vi "BioFeedback11(SingleBarBiofeedback).vi"(0 "UI Data Right":path=path "C:/Users/Tinggroup/Desktop/VRMuscleActivationVisualizer/VRBiofeedback_v2/assets/RightEMGData.txt", 7 "Frames Per Second":dbl=30.0, 9 "Start Trial":bool, 11 "End Trial":bool, 12 "Data Directory":path, 13 "File Name":string, 14 "Extension":string="_EMG.txt") -> ()   [LabVIEW 2016]
uses:
  <vilib>/Utility/error.llb/DialogType.ctl
  <vilib>/Analysis/5stat.llb/RMS (DBL).vi
  <vilib>/Waveform/WDTOps.llb/WDT Append Waveforms DBL.vi
  <vilib>/Utility/file.llb/Write Delimited Spreadsheet (string).vi
  <vilib>/Waveform/WDTFileIO.llb/Export Waveforms To Spreadsheet File (1D).vi
  <vilib>/Analysis/NI_AALPro.lvlib
panel:
  out "Trial Data Column Headers":string[](array[string])
  in  "TrialDataRowHeaders":string[](array[string])
  out "GetMaxStartTime":timestamp
  in  "SecondsToAcquireMax":dbl=10.0
  in  "NumberOfMaximumsInAverage":dbl=3.0
  in  "CurrentMaxIndex":dbl
  out "SignalsAvgMaxArray":dbl[](array[numeric])
  out "SignalMaxArray":dbl[][](array[numeric])
  in  "%StdDevIndex":dbl=5.0
  in  "Mean%Index":dbl=4.0
  in  "StdDevIndex":dbl=3.0
  in  "MeanIndex":dbl=2.0
  in  "MaxIndex":dbl=1.0
  in  "MinIndex":dbl
  out "Stability Data":dbl[][](array[numeric])
  out "2d target":cluster{dbl[], dbl[]}[](graph)
  out "trialFilteredData":waveform(dbl)[](array[waveform])
  out "filteredWaveforms":waveform(dbl)[](array[waveform])
  in  "UI Ampl Error Path":path=path "C:/Users/Tinggroup/Desktop/VRMuscleActivationVisualizer/VRBiofeedback_v2/assets/BiofeedbackAmplitudeError.txt"
  in  "UI L/R Error Path":path=path "C:/Users/Tinggroup/Desktop/VRMuscleActivationVisualizer/VRBiofeedback_v2/assets/BiofeedbackLRError.txt"
  out "LeftPercentActivation":dbl
  out "RightPercentActivation":dbl
  out "LeftMovingAvg":dbl
  out "RightMovingAvg":dbl
  in  "AutoAnalyzeStablity":bool
  out "PointCluster":cluster{dbl[], dbl[]}
  out "combined y value":dbl
  out "Acquiring Max":bool
  in  "resetMax":bool
  in  "startGetMax":bool
  in  "Right Max":dbl
  in  "Left Max":dbl
  in  "Amplitude Error":dbl
  in  "L/R error":dbl
  in  "RightSignalB":dbl=6.0
  in  "RightSignalA":dbl=5.0
  in  "LefftSignalB":dbl=2.0
  in  "LeftSignalA":dbl=1.0
  out "Aggregate 8":waveform(dbl)[](array[waveform])
  in  "UI Data Left":path=path "C:/Users/Tinggroup/Desktop/VRMuscleActivationVisualizer/VRBiofeedback_v2/assets/LeftEMGData.txt"
  in  "EMG Input Device\nProduct Type":string="USB-6009"
  out "DispLeftMovingAvg":dbl(slide) caption="Left" max=1.0 scale=0.0..100.0
  out "DispRightMovingAvg":dbl(slide) caption="Right" max=0.01 scale=0.0..100.0
  out "RMS Right":dbl(graph)
  out "RMS Left":dbl(graph)
  out "RMS 8":dbl(graph)
  out "RMS 7":dbl(graph)
  out "RMS 6":dbl(graph)
  out "RMS 5":dbl(graph)
  out "RMS 4":dbl(graph)
  out "RMS 3":dbl(graph)
  out "RMS 2":dbl(graph)
  out "RMS 1":dbl(graph)
  out "Aggregate7":waveform(dbl)[](array[waveform])
  out "Aggregate6":waveform(dbl)[](array[waveform])
  out "Aggregate5":waveform(dbl)[](array[waveform])
  out "Aggregate4":waveform(dbl)[](array[waveform])
  out "Aggregate3":waveform(dbl)[](array[waveform])
  out "Aggregate2":waveform(dbl)[](array[waveform])
  out "Aggregate1":waveform(dbl)[](array[waveform])
  out "Wfm8":waveform(dbl)(graph)
  out "Wfm7":waveform(dbl)(graph)
  out "Wfm6":waveform(dbl)(graph)
  out "Wfm5":waveform(dbl)(graph)
  out "Wfm4":waveform(dbl)(graph)
  out "Wfm3":waveform(dbl)(graph)
  out "Wfm2":waveform(dbl)(graph)
  out "Wfm1":waveform(dbl)(graph)
  out "Trial Raw Waveforms":waveform(dbl)[](graph)
  in  "UI Percent Path":path=path "C:/Users/Tinggroup/Desktop/VRMuscleActivationVisualizer/VRBiofeedback_v2/assets/BiofeedbackTargetPercentage.txt"
  in  "Target Percentage":dbl=10.0
  out "Trial In Progress":bool
  in  "Lower Cut-Off":dbl=20.0
  in  "Upper Cut-Off":dbl=300.0
  out "raw data":dynamicdata(graph)
  out "Bufffer Index":dbl
  out "Frames in Buffer":dbl
  out "Samples per frame":dbl
  out "Reset Data Acquisition\nAnd UI Updating":bool=TRUE
  in  "Moving Average Length (s)":dbl=0.5
  in  "Sample rate (Hz)":dbl=2000.0
  in  "End Program":bool
  # "Saving Trial Data"
  # "Set Target and Box Size"
  # "Set Scale"
  # "These scale the thermometers and are used in mean calculation"
  # "Analyze Stability of Displayed Data"
  # "Auto Analyze Stability begins calculating stability\nAs soon as dot enters the target zone and stops \nonce the dot leaves the target zone (Not Yet Implemented)"
  # "Channels used in Display"
  # "Filter and Process Parameters"
  # "Changes are made instantly and cause moving average to reset to zero"
  # "for testing smaller sample\nsizes in getting max/min\nand stability data"
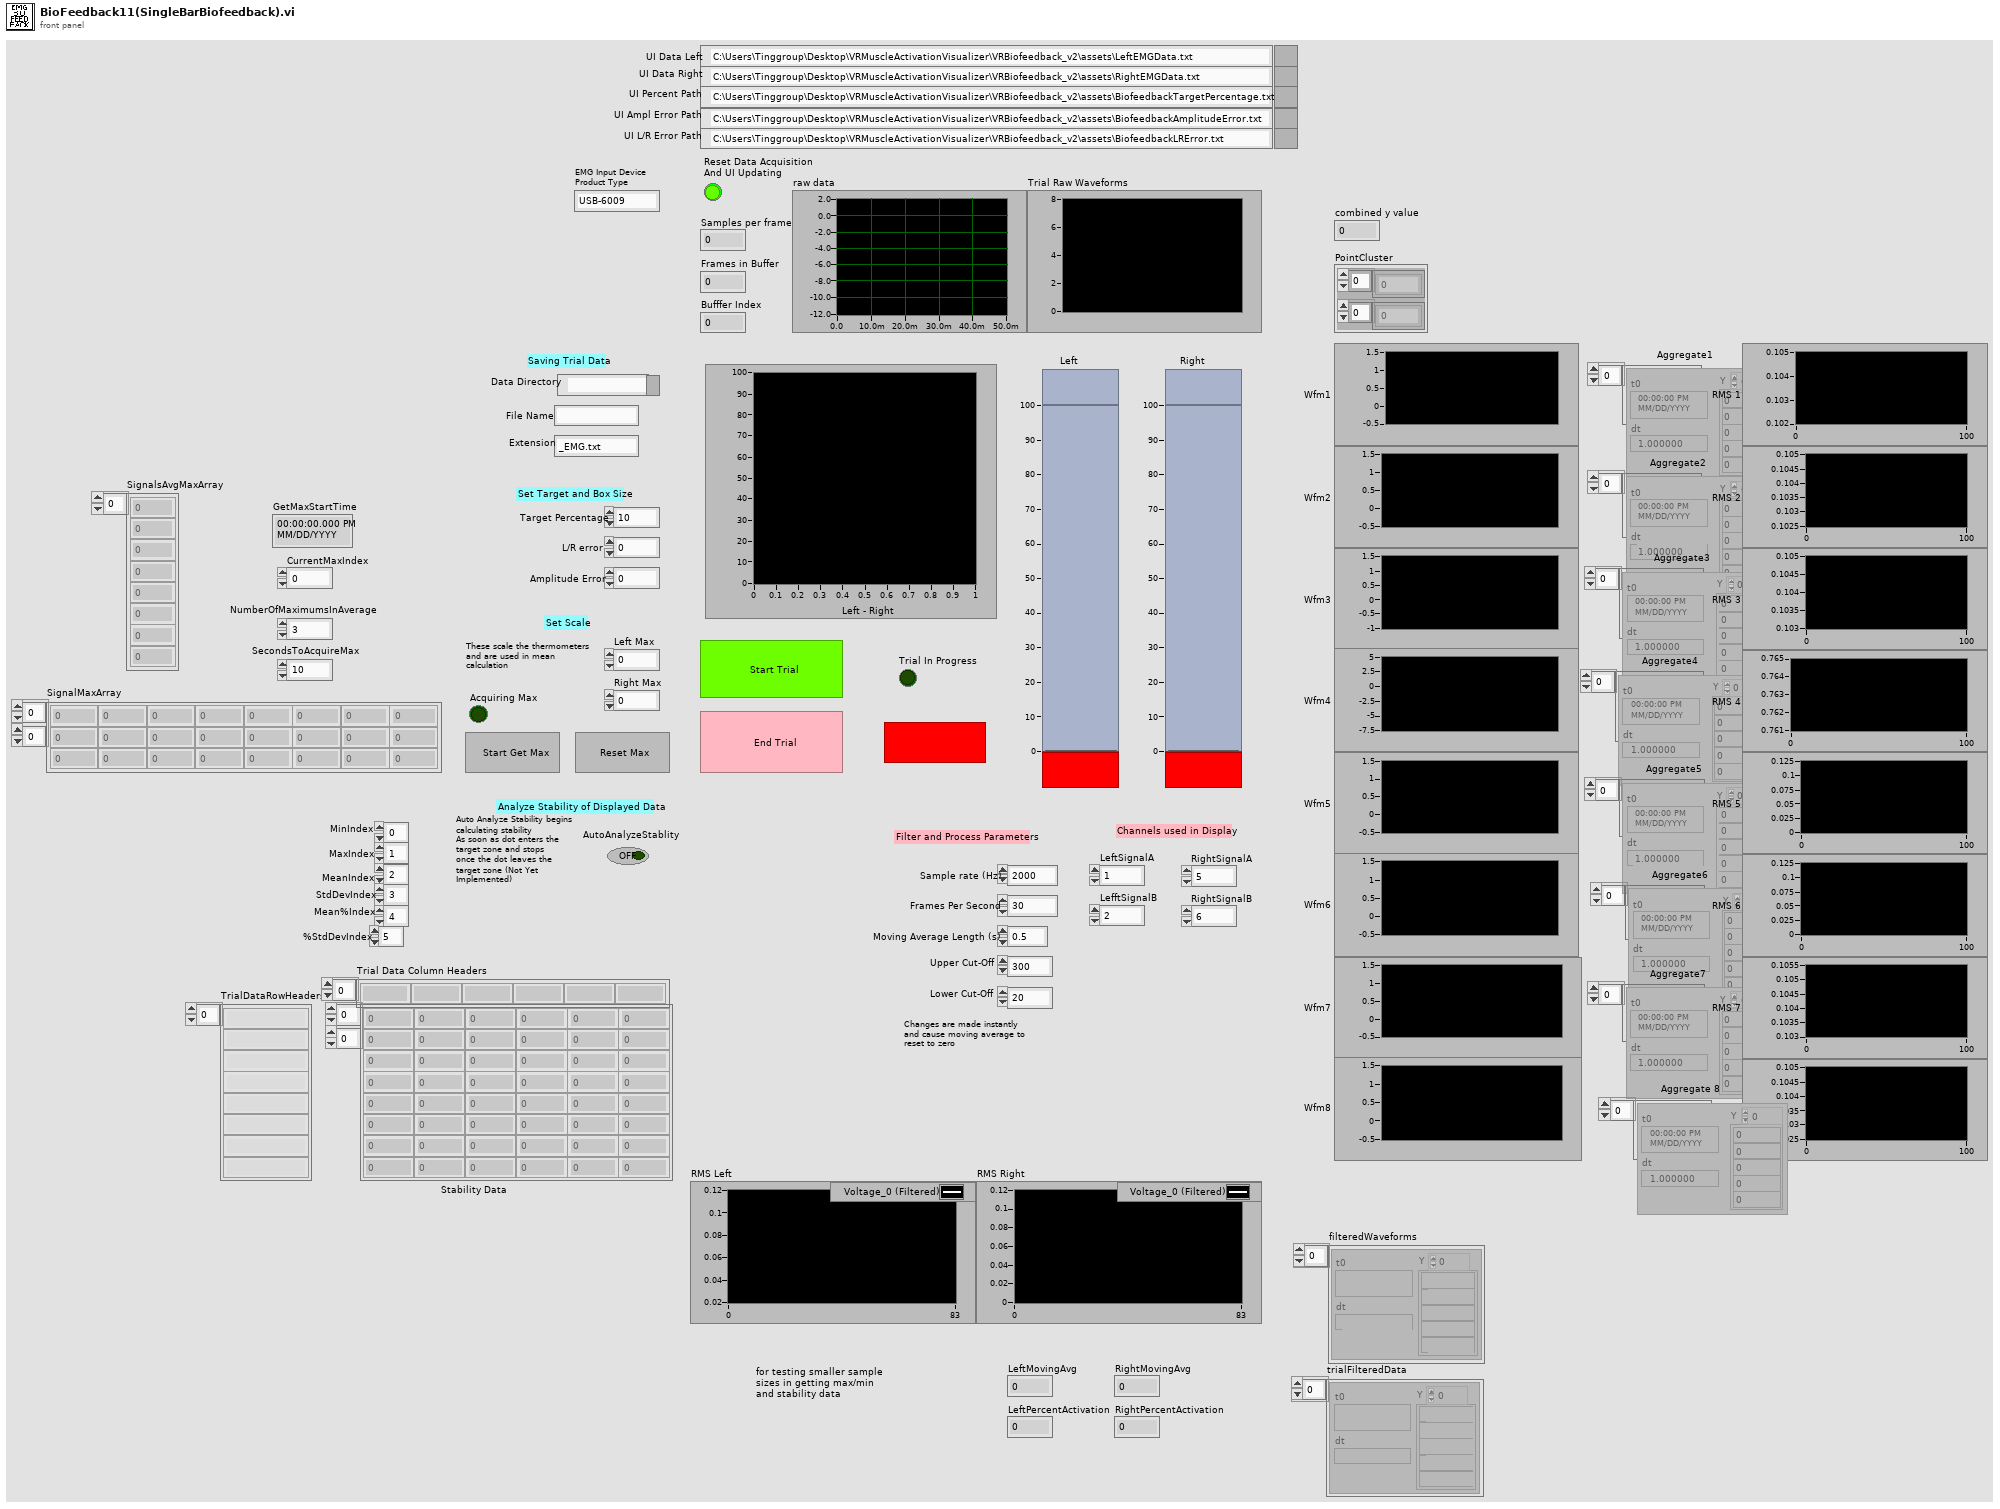
[diagram p1: front panel]
types:
  T1 = typedef "DialogType.ctl" = u16
  T2 = typedef "WaveformArrayControl.ctl" = waveform(dbl)[]
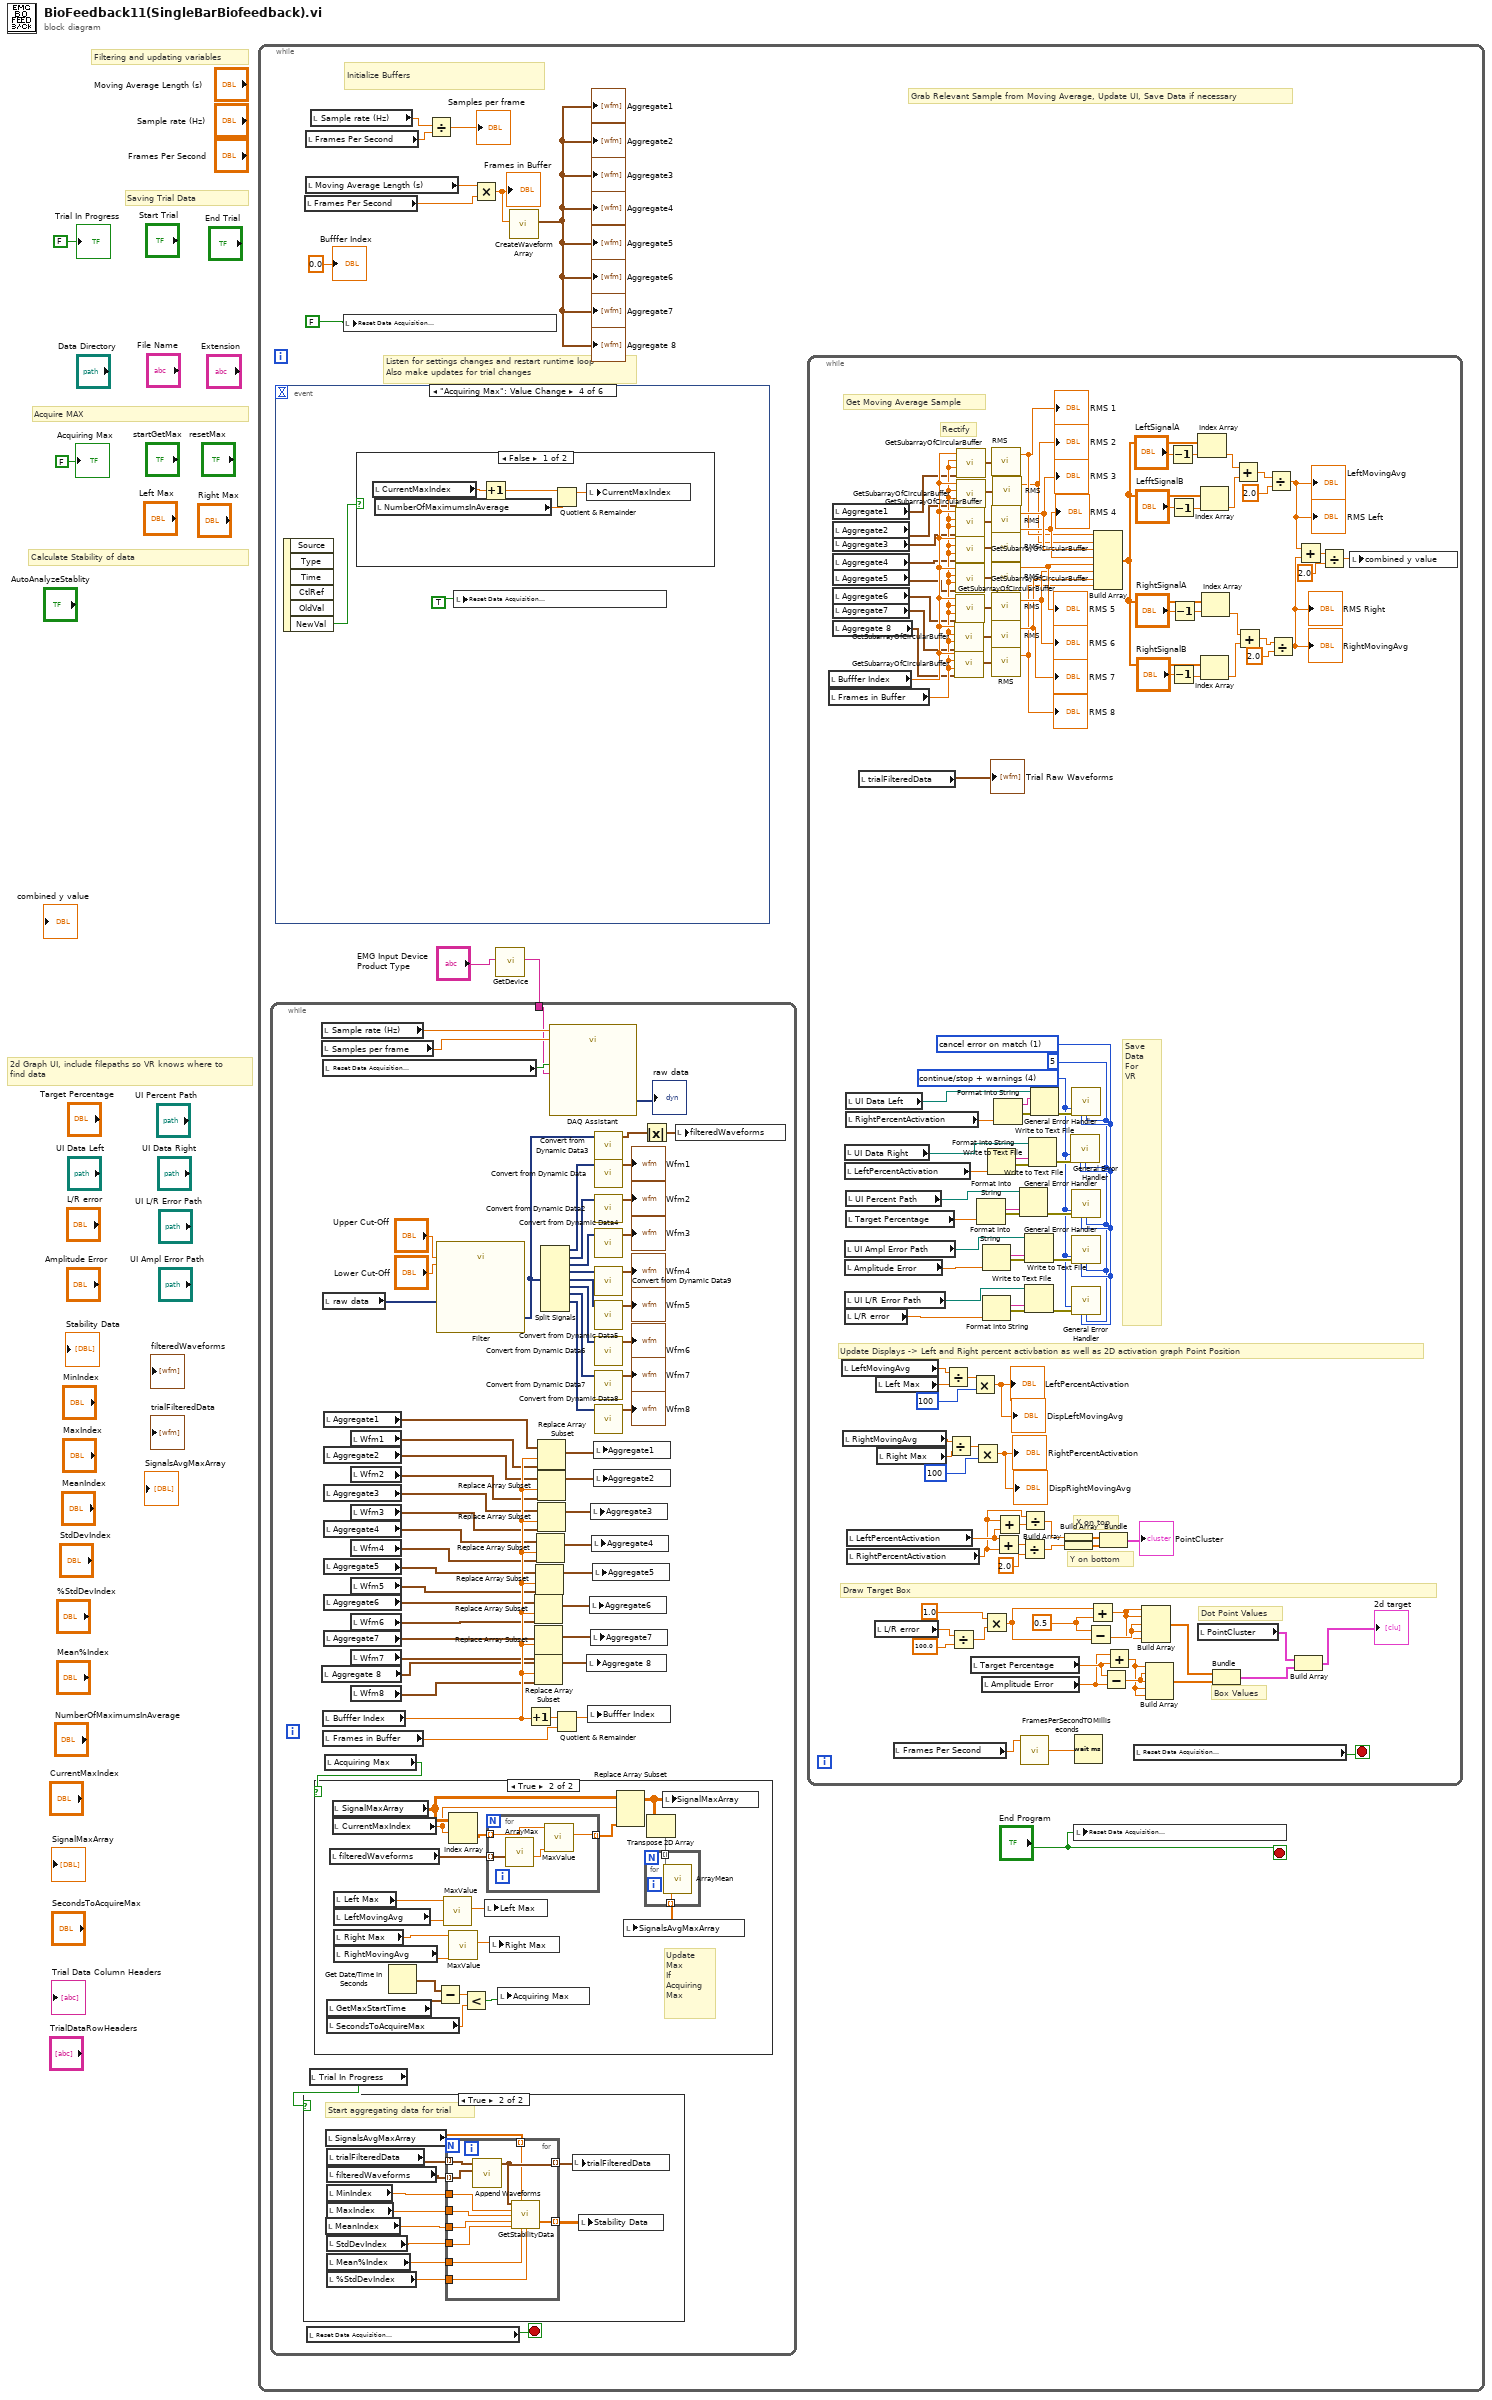
[diagram p0: block diagram]
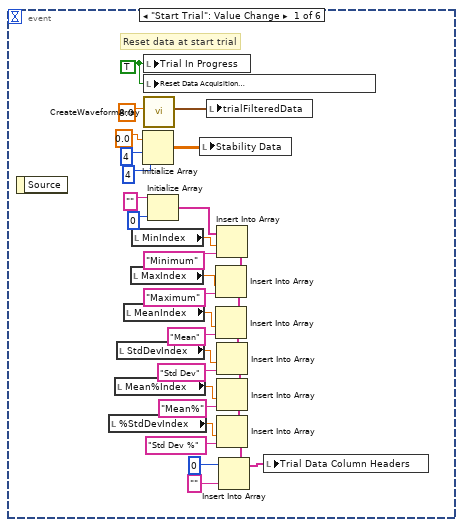
[diagram p2: hidden frame]
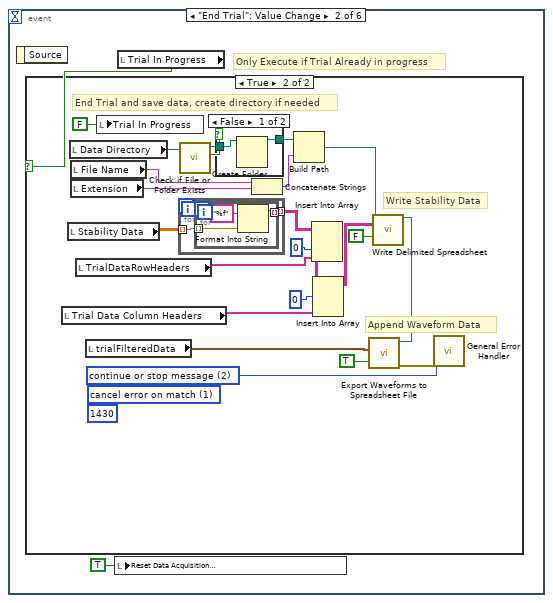
[diagram p3: hidden frame]
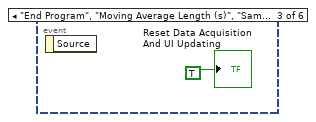
[diagram p6: hidden frame]
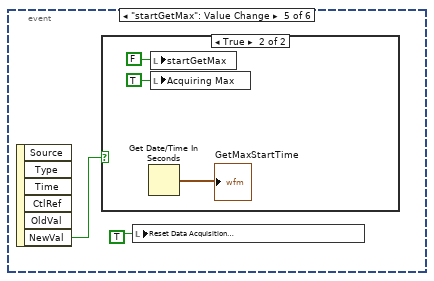
[diagram p8: hidden frame]
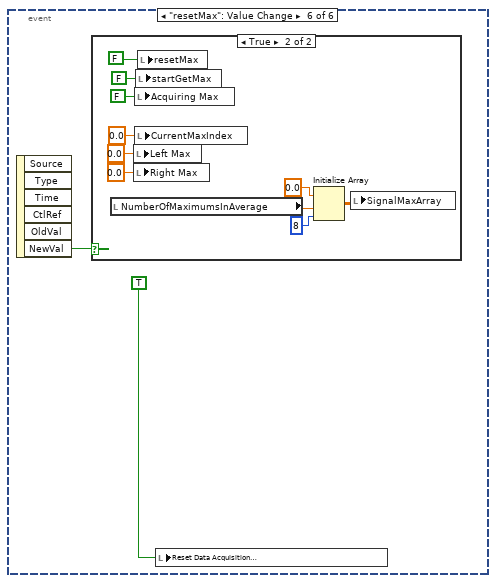
[diagram p10: hidden frame]
diagram:
  # "Calculate Stability of data"
  # "Acquire MAX"
  # "Filtering and updating variables"
  # "Saving Trial Data"
  # "2d Graph UI, include filepaths so VR knows where to find data"
  n1 = while {
    stop <- "End Program" stop-if-true
    # "Grab Relevant Sample from Moving Average, Update UI, Save Data if necessary"
    # "Initialize Buffers"
    # "Listen for settings changes and restart runtime loop\nAlso make updates for trial changes"
    n2 = event shown="[3] \"Acquiring Max\": Value Change" {
      selector: _ -> [_ _ _ _ _ _]
      dyn-events: _ -> [_ _ _ _ _ _]
      timeout: _ -> [_ _ _ _ _ _]
      event "Start Trial": Value Change {
        w45 = TRUE ("Trial In Progress")
        # "Reset data at start trial"
        n3 = event-data() -> ()  [unwired: 1 in, 1 out]
        n4 = local read "%StdDevIndex"() -> (w21:dbl)
        n5 = local read "Mean%Index"() -> (w22:dbl)
        n6 = local read "StdDevIndex"() -> (w26:dbl)
        n7 = local read "MeanIndex"() -> (w30:dbl)
        n8 = local read "MaxIndex"() -> (w33:dbl)
        n9 = local read "MinIndex"() -> (w35:dbl)
        n10 = Initialize Array(0.0 ("element"), 4 ("dimension size"), 4 ("dimension size")) -> (w39:dbl[][])
        n11 = local write "Trial In Progress"(w45) -> ()
        n12 = local write "Reset Data Acquisition\nAnd UI Updating"(w45) -> ()
        n13 = call "CreateWaveformArray.vi"("bufferSize"=8.0) -> ("initialized array"=w44:waveform(dbl)[])  [unwired: 5 in, 1 out]
        n14 = Initialize Array("", 0 ("dimension size")) -> (w34:string[])
        n15 = local write "Stability Data"(w39) -> ()
        n16 = local write "trialFilteredData"(w44) -> ()
        n17 = Insert Into Array(array=w34, index=w35, new element="Minimum" ("new element/subarray")) -> (w31:string[])
        n18 = Insert Into Array(array=w31, index=w33, new element="Maximum" ("new element/subarray")) -> (w28:string[])
        n19 = Insert Into Array(array=w28, index=w30, new element="Mean" ("new element/subarray")) -> (w25:string[])
        n20 = Insert Into Array(array=w25, index=w26, new element="Std Dev" ("new element/subarray")) -> (w23:string[])
        n21 = Insert Into Array(array=w23, index=w22, new element="Mean%" ("new element/subarray")) -> (w19:string[])
        n22 = Insert Into Array(array=w19, index=w21, new element="Std Dev %" ("new element/subarray")) -> (w16:string[])
        n23 = Insert Into Array(array=w16, index=0, new element="" ("new element/subarray")) -> (w17:string[])
        n24 = local write "Trial Data Column Headers"(w17) -> ()
      }
      event "End Trial": Value Change {
        # "Only Execute if Trial Already in progress"
        n25 = event-data() -> ()  [unwired: 1 in, 1 out]
        n26 = local write "Reset Data Acquisition\nAnd UI Updating"(TRUE ("Reset Data Acquisition\nAnd UI Updating")) -> ()
        n27 = local read "Trial In Progress"() -> (w47:bool)
        n28 = case shown="True" w47 {
          frame False {
          }
          frame True {
            w66 = T1 2 items=["no dialog", "OK message", "continue or stop message", "OK message + warnings", "continue/stop + warnings"] ("type of dialog (OK msg:1)")
            (unwired) 1 items=["no exception", "cancel error on match", "set error on match"] ("[exception action] (none:0)")
            (unwired) 1430 ("[exception code]")
            # "Append Waveform Data"
            # "Write Stability Data"
            # "End Trial and save data, create directory if needed"
            n29 = local read "Trial Data Column Headers"() -> (w54:string[])
            n30 = local read "Stability Data"() -> (w50:dbl[][])
            n31 = local read "Data Directory"() -> (w67:path)
            n32 = local read "File Name"() -> (w63:string)
            n33 = local read "Extension"() -> (w64:string)
            n34 = local read "TrialDataRowHeaders"() -> (w53:string[])
            n35 = local read "trialFilteredData"() -> (w56:waveform(dbl)[])
            n36 = local write "Trial In Progress"(FALSE ("Trial In Progress")) -> ()
            n37 = for {
              tunnel: w50 -> [w72] mode=indexing
              tunnel: [w71] -> w48 mode=indexing
              n38 = for {
                tunnel: w72 -> [w74] mode=indexing
                tunnel: [w73] -> w71 mode=indexing
                n39 = Format Into String(format string="%f", w74) -> (resulting string=w73:string)  [unwired: 2 in, 1 out]
              }
            }
            n40 = call <vilib>:"Check if File or Folder Exists.vi"("path"=w67) -> ("file or folder exists?"=w69:bool, "dup path"=w68:path)  [unwired: 8 in, 1 out]
            n41 = case shown="False" w69 {
              tunnel: [w76 w78] -> w65
              tunnel: w68 -> [w77 w78]
              frame False {
                n42 = Create Folder(path (use dialog)=w77) -> (created path=w76:path)  [unwired: 2 in, 2 out]
              }
              frame True {
              }
            }
            n43 = Concatenate Strings(w63, w64) -> (w62:string)
            n44 = Build Path(base path=w65, name or relative path=w62) -> (appended path=w59:path)
            n45 = Insert Into Array(array=w48, index (col)=0 ("index (row)"), new element=w53) -> (w60:string[][])  [unwired: 1 in]
            n46 = Insert Into Array(array=w60, index (row)=0 ("index (col)"), new element=w54) -> (w49:string[][])  [unwired: 1 in]
            n47 = call-poly <vilib>:"Write Delimited Spreadsheet.vi"("file path (dialog if empty)"=w59, "2D data"=w49, "append to file? (new file:F)"=FALSE) -> ("new file path (Not A Path if cancelled)"=w57:path)  [unwired: 11 in, 1 out]
            n48 = call-poly <vilib>:"Export Waveforms to Spreadsheet File.vi"("append to file? (new file:F)"=TRUE, "waveforms"=w56, "file path (dialog if empty)"=w57) -> ("error out"=w61:errorcluster)  [unwired: 7 in, 1 out]
            n49 = call <vilib>:"General Error Handler.vi"("type of dialog (OK msg:1)"=w66, "error in (no error)"=w61) -> ()  [unwired: 9 in, 5 out]
          }
        }
      }
      event "End Program", "Moving Average Length (s)", "Sample rate (Hz)", "Frames Per Second": Value Change {
        n50 = event-data() -> ()  [unwired: 1 in, 1 out]
        "Reset Data Acquisition\nAnd UI Updating" <- TRUE
      }
      event "Acquiring Max": Value Change {
        n51 = event-data() -> ("NewVal"=w81:bool)  [unwired: 1 in, 5 out]
        n52 = case shown="False" w81 {
          frame False {
            n53 = local read "CurrentMaxIndex"() -> (w85:dbl)
            n54 = local read "NumberOfMaximumsInAverage"() -> (w83:dbl)
            n55 = Increment(x=w85) -> (x+1=w84:dbl)
            n56 = Quotient & Remainder(x=w84, y=w83) -> (x-y*floor(x/y)=w82:dbl)  [unwired: 1 out]
            n57 = local write "CurrentMaxIndex"(w82) -> ()
          }
          frame True {
          }
        }
        n58 = local write "Reset Data Acquisition\nAnd UI Updating"(TRUE ("Reset Data Acquisition\nAnd UI Updating")) -> ()
      }
      event "startGetMax": Value Change {
        n59 = event-data() -> ("NewVal"=w87:bool)  [unwired: 1 in, 5 out]
        n60 = case shown="True" w87 {
          frame False {
          }
          frame True {
            n61 = Get Date/Time In Seconds() -> (seconds since 1Jan1904=→"GetMaxStartTime":timestamp)
            n62 = local write "startGetMax"(FALSE) -> ()
            n63 = local write "Acquiring Max"(TRUE ("Acquiring Max")) -> ()
          }
        }
        n64 = local write "Reset Data Acquisition\nAnd UI Updating"(TRUE ("Reset Data Acquisition\nAnd UI Updating")) -> ()
      }
      event "resetMax": Value Change {
        n65 = event-data() -> ("NewVal"=w92:bool)  [unwired: 1 in, 5 out]
        n66 = case shown="True" w92 {
          frame False {
          }
          frame True {
            n67 = local read "NumberOfMaximumsInAverage"() -> (w95:dbl)
            n68 = local write "Left Max"(0.0 ("Left Max")) -> ()
            n69 = local write "Right Max"(0.0 ("Right Max")) -> ()
            n70 = local write "Acquiring Max"(FALSE ("Acquiring Max")) -> ()
            n71 = local write "CurrentMaxIndex"(0.0 ("CurrentMaxIndex")) -> ()
            n72 = local write "startGetMax"(FALSE ("startGetMax")) -> ()
            n73 = local write "resetMax"(FALSE ("endGetMax")) -> ()
            n74 = Initialize Array(0.0 ("element"), w95, 8 ("dimension size")) -> (w96:dbl[][])
            n75 = local write "SignalMaxArray"(w96) -> ()
          }
        }
        n76 = local write "Reset Data Acquisition\nAnd UI Updating"(TRUE ("Reset Data Acquisition\nAnd UI Updating")) -> ()
      }
    }
    n77 = local read "Frames Per Second"() -> (w10:dbl)
    n78 = local read "Frames Per Second"() -> (w13:dbl)
    n79 = local read "Moving Average Length (s)"() -> (w11:dbl)
    n80 = local read "Sample rate (Hz)"() -> (w14:dbl)
    n81 = local write "Reset Data Acquisition\nAnd UI Updating"(FALSE) -> ()
    n82 = Divide(x=w14, y=w13) -> (x/y=→"Samples per frame":dbl)
    n83 = Multiply(x=w11, y=w10) -> (x*y=w7:dbl)
    "Frames in Buffer" <- w7
    n84 = call "GetDevice.vi"("EMG Input Device\nProduct Type"="EMG Input Device\nProduct Type") -> ("DAQmx Device Name"=w3:tag)  [unwired: 10 in]
    n85 = while {
      tunnel: w3 -> [w223]
      stop <- w270 stop-if-true
      n86 = local read "Reset Data Acquisition\nAnd UI Updating"() -> (w270:bool)
      n87 = local read "Trial In Progress"() -> (w228:bool)
      n88 = case shown="True" w228 {
        frame False {
        }
        frame True {
          # "Start aggregating data for trial"
          n89 = local read "SignalsAvgMaxArray"() -> (w305:dbl[])
          n90 = local read "MeanIndex"() -> (w309:dbl)
          n91 = local read "trialFilteredData"() -> (w312:waveform(dbl)[])
          n92 = local read "filteredWaveforms"() -> (w313:waveform(dbl)[])
          n93 = local read "MinIndex"() -> (w311:dbl)
          n94 = local read "MaxIndex"() -> (w310:dbl)
          n95 = local read "StdDevIndex"() -> (w308:dbl)
          n96 = local read "Mean%Index"() -> (w307:dbl)
          n97 = local read "%StdDevIndex"() -> (w306:dbl)
          n98 = for {
            tunnel: w313 -> [w323] mode=indexing
            tunnel: w312 -> [w324] mode=indexing
            tunnel: [w322] -> w303 mode=indexing
            tunnel: [w314] -> w304 mode=indexing
            tunnel: w311 -> [w321]
            tunnel: w310 -> [w320]
            tunnel: w309 -> [w319]
            tunnel: w308 -> [w318]
            tunnel: w307 -> [w317]
            tunnel: w306 -> [w316]
            tunnel: w305 -> [w315] mode=indexing
            n99 = call-poly <vilib>:"Append Waveforms.vi"("waveform B"=w323, "waveform A"=w324) -> ("waveform out"=w322:waveform(dbl))  [unwired: 8 in, 1 out]
            n100 = call "GetStabilityData.vi"("ProvidedData"=w322, "ScaleMax"=w315, "MinIndex"=w321, "MaxIndex"=w320, "MeanIndex"=w319, "StdDevIndex"=w318, "Mean%Index"=w317, "%StdDevIndex"=w316) -> ("ReturnData"=w314:dbl[])  [unwired: 7 in]
          }
          n101 = local write "trialFilteredData"(w303) -> ()
          n102 = local write "Stability Data"(w304) -> ()
        }
      }
      n103 = local read "Sample rate (Hz)"() -> (w277:dbl)
      n104 = local read "Samples per frame"() -> (w276:dbl)
      n105 = local read "Aggregate 8"() -> (w226:waveform(dbl)[])
      n106 = local read "Reset Data Acquisition\nAnd UI Updating"() -> (w269:bool)
      n107 = local read "raw data"() -> (w275:dynamicdata)
      n108 = local read "Bufffer Index"() -> (w251:dbl)
      n109 = local read "Frames in Buffer"() -> (w272:dbl)
      n110 = local read "Aggregate1"() -> (w250:waveform(dbl)[])
      n111 = local read "Aggregate2"() -> (w248:waveform(dbl)[])
      n112 = local read "Aggregate3"() -> (w246:waveform(dbl)[])
      n113 = local read "Aggregate4"() -> (w244:waveform(dbl)[])
      n114 = local read "Aggregate5"() -> (w242:waveform(dbl)[])
      n115 = local read "Aggregate6"() -> (w240:waveform(dbl)[])
      n116 = local read "Aggregate7"() -> (w238:waveform(dbl)[])
      n117 = local read "Acquiring Max"() -> (w220:bool)
      n118 = case shown="True" w220 {
        frame False {
        }
        frame True {
          # "Update\nMax\nIf \nAcquiring\nMax"
          n119 = local read "GetMaxStartTime"() -> (w285:timestamp)
          n120 = local read "SecondsToAcquireMax"() -> (w282:dbl)
          n121 = local read "filteredWaveforms"() -> (w295:waveform(dbl)[])
          n122 = local read "SignalMaxArray"() -> (w288:dbl[][])
          n123 = local read "CurrentMaxIndex"() -> (w287:dbl)
          n124 = local read "Left Max"() -> (w294:dbl)
          n125 = local read "LeftMovingAvg"() -> (w293:dbl)
          n126 = local read "Right Max"() -> (w291:dbl)
          n127 = local read "RightMovingAvg"() -> (w290:dbl)
          n128 = Get Date/Time In Seconds() -> (seconds since 1Jan1904=w284:timestamp)
          n129 = Subtract(x=w284, y=w285) -> (x-y=w283:dbl)
          n130 = call "MaxValue.vi"("NewValue"=w293, "CurrentMax"=w294) -> ("Max"=w292:dbl)  [unwired: 9 in]
          n131 = Index Array(array=w288, index (row)=w287) -> (element=w296:dbl[])  [unwired: 1 in]
          n132 = call "MaxValue.vi"("NewValue"=w290, "CurrentMax"=w291) -> ("Max"=w289:dbl)  [unwired: 9 in]
          n133 = Less?(x=w283, y=w282) -> (x < y?=w281:bool)
          n134 = local write "Left Max"(w292) -> ()
          n135 = for {
            tunnel: w296 -> [w300] mode=indexing
            tunnel: w295 -> [w302] mode=indexing
            tunnel: [w299] -> w286 mode=indexing
            n136 = call "ArrayMax.vi"("Array"=w302) -> ("max"=w301:dbl)  [unwired: 10 in]
            n137 = call "MaxValue.vi"("NewValue"=w301, "CurrentMax"=w300) -> ("Max"=w299:dbl)  [unwired: 9 in]
          }
          n138 = local write "Right Max"(w289) -> ()
          n139 = local write "Acquiring Max"(w281) -> ()
          n140 = Replace Array Subset(array=w288, new element=w286, index (row)=w287) -> (w280:dbl[][])  [unwired: 1 in]
          n141 = Transpose 2D Array(2D array=w280) -> (transposed array=w279:dbl[][])
          n142 = for {
            tunnel: w279 -> [w298] mode=indexing
            tunnel: [w297] -> w278 mode=indexing
            n143 = call "ArrayMean.vi"("Array"=w298) -> ("Mean"=w297:dbl)  [unwired: 10 in]
          }
          n144 = local write "SignalsAvgMaxArray"(w278) -> ()
          n145 = local write "SignalMaxArray"(w280) -> ()
        }
      }
      n146 = local read "Wfm1"() -> (w249:waveform(dbl))
      n147 = local read "Wfm2"() -> (w247:waveform(dbl))
      n148 = local read "Wfm3"() -> (w245:waveform(dbl))
      n149 = local read "Wfm4"() -> (w243:waveform(dbl))
      n150 = local read "Wfm5"() -> (w241:waveform(dbl))
      n151 = local read "Wfm6"() -> (w239:waveform(dbl))
      n152 = local read "Wfm7"() -> (w237:waveform(dbl))
      n153 = local read "Wfm8"() -> (w236:waveform(dbl))
      n154 = call "Filter"("Lower Cut-Off"="Lower Cut-Off", "Upper Cut-Off"="Upper Cut-Off", "Signal"=w275) -> ("Filtered Signal"=w224:dynamicdata)  [unwired: 7 in, 1 out]
      n155 = Increment(x=w251) -> (x+1=w271:dbl)
      n156 = Replace Array Subset(array=w240, new element=w239, index=w251) -> (w230:waveform(dbl)[])
      n157 = Replace Array Subset(array=w238, new element=w237, index=w251) -> (w229:waveform(dbl)[])
      n158 = Replace Array Subset(array=w226, new element=w236, index=w251) -> (w227:waveform(dbl)[])
      n159 = Replace Array Subset(array=w242, new element=w241, index=w251) -> (w231:waveform(dbl)[])
      n160 = Replace Array Subset(array=w244, new element=w243, index=w251) -> (w232:waveform(dbl)[])
      n161 = Replace Array Subset(array=w250, new element=w249, index=w251) -> (w235:waveform(dbl)[])
      n162 = Replace Array Subset(array=w248, new element=w247, index=w251) -> (w234:waveform(dbl)[])
      n163 = Replace Array Subset(array=w246, new element=w245, index=w251) -> (w233:waveform(dbl)[])
      n164 = Split Signals(w224) -> (w267:dynamicdata, w266:dynamicdata, w265:dynamicdata, w264:dynamicdata, w263:dynamicdata, w262:dynamicdata, w261:dynamicdata, w260:dynamicdata)  [unwired: 9 in, 1 out]
      n165 = call "DAQ Assistant"("rate"=w277, "number of samples"=w276, "stop (T)"=w269, "device name"=w223) -> ("data"=→"raw data":dynamicdata)  [unwired: 13 in, 2 out]
      n166 = Quotient & Remainder(x=w271, y=w272) -> (x-y*floor(x/y)=w273:dbl)  [unwired: 1 out]
      n167 = local write "Aggregate 8"(w227) -> ()
      n168 = local write "Bufffer Index"(w273) -> ()
      n169 = local write "Aggregate6"(w230) -> ()
      n170 = local write "Aggregate3"(w233) -> ()
      n171 = local write "Aggregate7"(w229) -> ()
      n172 = local write "Aggregate4"(w232) -> ()
      n173 = local write "Aggregate5"(w231) -> ()
      n174 = local write "Aggregate1"(w235) -> ()
      n175 = local write "Aggregate2"(w234) -> ()
      n176 = call "Convert from Dynamic Data3"("Dynamic Data Type"=w224) -> ("Array of Waveform"=w222:waveform(dbl)[])  [unwired: 3 in]
      n177 = call "Convert from Dynamic Data"("Dynamic Data Type"=w267) -> ("Waveform"=→"Wfm1":waveform(dbl))  [unwired: 3 in]
      n178 = call "Convert from Dynamic Data2"("Dynamic Data Type"=w266) -> ("Waveform"=→"Wfm2":waveform(dbl))  [unwired: 3 in]
      n179 = call "Convert from Dynamic Data4"("Dynamic Data Type"=w265) -> ("Waveform"=→"Wfm3":waveform(dbl))  [unwired: 3 in]
      n180 = call "Convert from Dynamic Data9"("Dynamic Data Type"=w264) -> ("Waveform"=→"Wfm4":waveform(dbl))  [unwired: 3 in]
      n181 = call "Convert from Dynamic Data5"("Dynamic Data Type"=w263) -> ("Waveform"=→"Wfm5":waveform(dbl))  [unwired: 3 in]
      n182 = call "Convert from Dynamic Data6"("Dynamic Data Type"=w262) -> ("Waveform"=→"Wfm6":waveform(dbl))  [unwired: 3 in]
      n183 = call "Convert from Dynamic Data7"("Dynamic Data Type"=w261) -> ("Waveform"=→"Wfm7":waveform(dbl))  [unwired: 3 in]
      n184 = call "Convert from Dynamic Data8"("Dynamic Data Type"=w260) -> ("Waveform"=→"Wfm8":waveform(dbl))  [unwired: 3 in]
      n185 = Absolute Value(x=w222) -> (abs(x)=w221:waveform(dbl)[])
      n186 = local write "filteredWaveforms"(w221) -> ()
    }
    n187 = call "CreateWaveformArray.vi"("bufferSize"=w7) -> ("initialized array"=→"Aggregate1" →"Aggregate2" →"Aggregate3" →"Aggregate4" →"Aggregate5" →"Aggregate6" →"Aggregate7" →"Aggregate 8":waveform(dbl)[])  [unwired: 5 in, 1 out]
    n188 = while {
      stop <- w219 stop-if-true
      w162 = 0.5 ("element")
      w117 = T1 4 items=["no dialog", "OK message", "continue or stop message", "OK message + warnings", "continue/stop + warnings"] ("type of dialog (OK msg:1)")
      w116 = 1 items=["no exception", "cancel error on match", "set error on match"] ("[exception action] (none:0)")
      w115 = 5 ("[exception code]")
      # "Y on bottom"
      # "X on top"
      # "Dot Point Values"
      # "Box Values"
      # "Update Displays -> Left and Right percent activbation as well as 2D activation graph Point Position"
      # "Draw Target Box"
      # "Save\nData\nFor\nVR"
      # "Get Moving Average Sample"
      # "Rectify"
      n189 = local read "Bufffer Index"() -> (w211:dbl)
      n190 = local read "Frames in Buffer"() -> (w210:dbl)
      n191 = local read "Aggregate1"() -> (w209:waveform(dbl)[])
      n192 = local read "Aggregate2"() -> (w205:waveform(dbl)[])
      n193 = local read "Aggregate3"() -> (w208:waveform(dbl)[])
      n194 = local read "Aggregate4"() -> (w204:waveform(dbl)[])
      n195 = local read "Aggregate5"() -> (w207:waveform(dbl)[])
      n196 = local read "Aggregate6"() -> (w206:waveform(dbl)[])
      n197 = local read "Aggregate7"() -> (w203:waveform(dbl)[])
      n198 = local read "Aggregate 8"() -> (w192:waveform(dbl)[])
      n199 = local read "LeftMovingAvg"() -> (w146:dbl)
      n200 = local read "RightMovingAvg"() -> (w142:dbl)
      n201 = local read "UI Data Right"() -> (w215:path)
      n202 = local read "LeftPercentActivation"() -> (w213:dbl)
      n203 = local read "UI Ampl Error Path"() -> (w118:path)
      n204 = local read "Amplitude Error"() -> (w119:dbl)
      n205 = local read "UI L/R Error Path"() -> (w121:path)
      n206 = local read "L/R error"() -> (w120:dbl)
      n207 = local read "UI Data Left"() -> (w200:path)
      n208 = local read "RightPercentActivation"() -> (w202:dbl)
      n209 = local read "UI Percent Path"() -> (w194:path)
      n210 = local read "Target Percentage"() -> (w193:dbl)
      n211 = local read "LeftPercentActivation"() -> (w135:dbl)
      n212 = local read "RightPercentActivation"() -> (w133:dbl)
      n213 = local read "trialFilteredData"() -> (→"Trial Raw Waveforms":waveform(dbl)[])
      n214 = local read "L/R error"() -> (w173:dbl)
      n215 = local read "Left Max"() -> (w145:dbl)
      n216 = local read "Right Max"() -> (w141:dbl)
      n217 = local read "Frames Per Second"() -> (w218:dbl)
      n218 = Divide(x=w146, y=w145) -> (x/y=w147:dbl)
      n219 = Divide(x=w142, y=w141) -> (x/y=w143:dbl)
      n220 = Divide(x=w173, y=100.0) -> (x/y=w167:dbl)
      n221 = call "GetSubarrayOfCircularBuffer.vi"("initialized array"=w203, "buffer size"=w210, "subset size"=w210, "start index"=w211) -> ("initialized array 2"=w104:T2)  [unwired: 7 in]
      n222 = call "GetSubarrayOfCircularBuffer.vi"("initialized array"=w192, "buffer size"=w210, "subset size"=w210, "start index"=w211) -> ("initialized array 2"=w103:T2)  [unwired: 7 in]
      n223 = call "GetSubarrayOfCircularBuffer.vi"("initialized array"=w208, "buffer size"=w210, "subset size"=w210, "start index"=w211) -> ("initialized array 2"=w108:T2)  [unwired: 7 in]
      n224 = call "GetSubarrayOfCircularBuffer.vi"("initialized array"=w204, "buffer size"=w210, "subset size"=w210, "start index"=w211) -> ("initialized array 2"=w107:T2)  [unwired: 7 in]
      n225 = call "GetSubarrayOfCircularBuffer.vi"("initialized array"=w207, "buffer size"=w210, "subset size"=w210, "start index"=w211) -> ("initialized array 2"=w106:T2)  [unwired: 7 in]
      n226 = call "GetSubarrayOfCircularBuffer.vi"("initialized array"=w206, "buffer size"=w210, "subset size"=w210, "start index"=w211) -> ("initialized array 2"=w105:T2)  [unwired: 7 in]
      n227 = call "GetSubarrayOfCircularBuffer.vi"("initialized array"=w209, "buffer size"=w210, "subset size"=w210, "start index"=w211) -> ("initialized array 2"=w110:T2)  [unwired: 7 in]
      n228 = call "GetSubarrayOfCircularBuffer.vi"("initialized array"=w205, "buffer size"=w210, "subset size"=w210, "start index"=w211) -> ("initialized array 2"=w109:T2)  [unwired: 7 in]
      n229 = Multiply(x=w147, y=100) -> (x*y=→"DispLeftMovingAvg" →"LeftPercentActivation":dbl)
      n230 = local read "Target Percentage"() -> (w114:dbl)
      n231 = Multiply(x=w143, y=100) -> (x*y=→"DispRightMovingAvg" →"RightPercentActivation":dbl)
      n232 = Format Into String(w193) -> (resulting string=w195:string, error out=w196:errorcluster)  [unwired: 3 in]
      n233 = local read "Amplitude Error"() -> (w113:dbl)
      n234 = Format Into String(w119) -> (resulting string=w125:string, error out=w126:errorcluster)  [unwired: 3 in]
      n235 = Format Into String(w120) -> (resulting string=w122:string, error out=w123:errorcluster)  [unwired: 3 in]
      n236 = Multiply(x=1.0, y=w167) -> (x*y=w166:dbl)
      n237 = Format Into String(w213) -> (resulting string=w214:string, error out=w216:errorcluster)  [unwired: 3 in]
      n238 = call-poly <vilib>:"RMS.vi"("X"=w110) -> ("rms value"=w186:dbl)  [unwired: 1 out]
      "RMS 1" <- w186
      n239 = call-poly <vilib>:"RMS.vi"("X"=w108) -> ("rms value"=w191:dbl)  [unwired: 1 out]
      "RMS 3" <- w191
      n240 = call-poly <vilib>:"RMS.vi"("X"=w107) -> ("rms value"=w190:dbl)  [unwired: 1 out]
      "RMS 4" <- w190
      n241 = call-poly <vilib>:"RMS.vi"("X"=w106) -> ("rms value"=w189:dbl)  [unwired: 1 out]
      "RMS 5" <- w189
      n242 = call-poly <vilib>:"RMS.vi"("X"=w105) -> ("rms value"=w188:dbl)  [unwired: 1 out]
      "RMS 6" <- w188
      n243 = call-poly <vilib>:"RMS.vi"("X"=w104) -> ("rms value"=w187:dbl)  [unwired: 1 out]
      "RMS 7" <- w187
      n244 = call-poly <vilib>:"RMS.vi"("X"=w103) -> ("rms value"=w184:dbl)  [unwired: 1 out]
      "RMS 8" <- w184
      n245 = call-poly <vilib>:"RMS.vi"("X"=w109) -> ("rms value"=w185:dbl)  [unwired: 1 out]
      "RMS 2" <- w185
      n246 = Format Into String(w202) -> (resulting string=w199:string, error out=w201:errorcluster)  [unwired: 3 in]
      n247 = Add(x=w135, y=w133) -> (x+y=w137:dbl)
      n248 = Add(x=w133, y=w135) -> (x+y=w134:dbl)
      n249 = Write to Text File(file (use dialog)=w194, text=w195, error in=w196) -> (error out=w197:errorcluster)  [unwired: 1 in, 2 out]
      n250 = Divide(x=w137, y=2.0) -> (x/y=w136:dbl)
      n251 = call "FramesPerSecondTOMilliseconds.vi"("Thermometer\nFps"=w218) -> ("x*y"=w111:dbl)  [unwired: 10 in]
      n252 = Divide(x=w133, y=w134) -> (x/y=w132:dbl)
      n253 = Write to Text File(file (use dialog)=w118, text=w125, error in=w126) -> (error out=w127:errorcluster)  [unwired: 1 in, 2 out]
      n254 = Write to Text File(file (use dialog)=w121, text=w122, error in=w123) -> (error out=w124:errorcluster)  [unwired: 1 in, 2 out]
      n255 = Write to Text File(file (use dialog)=w215, text=w214, error in=w216) -> (error out=w217:errorcluster)  [unwired: 1 in, 2 out]
      n256 = Write to Text File(file (use dialog)=w200, text=w199, error in=w201) -> (error out=w198:errorcluster)  [unwired: 1 in, 2 out]
      n257 = Build Array(w132) -> (w178:dbl[])
      n258 = Build Array(w136) -> (w176:dbl[])
      n259 = call <vilib>:"General Error Handler.vi"("type of dialog (OK msg:1)"=w117, "error in (no error)"=w217, "[exception action] (none:0)"=w116, "[exception code]"=w115) -> ()  [unwired: 7 in, 5 out]
      n260 = call <vilib>:"General Error Handler.vi"("type of dialog (OK msg:1)"=w117, "error in (no error)"=w198, "[exception action] (none:0)"=w116, "[exception code]"=w115) -> ()  [unwired: 7 in, 5 out]
      n261 = call <vilib>:"General Error Handler.vi"("type of dialog (OK msg:1)"=w117, "error in (no error)"=w197, "[exception action] (none:0)"=w116, "[exception code]"=w115) -> ()  [unwired: 7 in, 5 out]
      n262 = call <vilib>:"General Error Handler.vi"("type of dialog (OK msg:1)"=w117, "error in (no error)"=w127, "[exception action] (none:0)"=w116, "[exception code]"=w115) -> ()  [unwired: 7 in, 5 out]
      n263 = call <vilib>:"General Error Handler.vi"("type of dialog (OK msg:1)"=w117, "error in (no error)"=w124, "[exception action] (none:0)"=w116, "[exception code]"=w115) -> ()  [unwired: 7 in, 5 out]
      n264 = Wait (ms)(milliseconds to wait=w111) -> ()  [unwired: 1 out]
      n265 = Subtract(x=w162, y=w166) -> (x-y=w172:dbl)
      n266 = Add(x=w166, y=w162) -> (x+y=w168:dbl)
      n267 = Build Array(w186, w185, w191, w190, w189, w188, w187, w184) -> (w183:dbl[])
      n268 = Bundle(w178, w176) -> (→"PointCluster":cluster{dbl[], dbl[]})  [unwired: 1 in]
      n269 = Subtract(x=w114, y=w113) -> (x-y=w170:dbl)
      n270 = Add(x=w113, y=w114) -> (x+y=w169:dbl)
      n271 = local read "Reset Data Acquisition\nAnd UI Updating"() -> (w219:bool)
      n272 = Build Array(w168, w168, w172, w172, w168) -> (w164:dbl[])
      n273 = Build Array(w169, w170, w170, w169, w169) -> (w165:dbl[])
      n274 = Decrement(x="LeftSignalA") -> (x-1=w153:dbl)
      n275 = Decrement(x="LefftSignalB") -> (x-1=w155:dbl)
      n276 = Decrement(x="RightSignalB") -> (x-1=w151:dbl)
      n277 = Decrement(x="RightSignalA") -> (x-1=w149:dbl)
      n278 = Index Array(array=w183, index=w153) -> (element=w160:dbl)
      n279 = local read "PointCluster"() -> (w161:cluster{dbl[], dbl[]})
      n280 = Index Array(array=w183, index=w155) -> (element=w159:dbl)
      n281 = Index Array(array=w183, index=w151) -> (element=w181:dbl)
      n282 = Index Array(array=w183, index=w149) -> (element=w182:dbl)
      n283 = Bundle(w164, w165) -> (w171:cluster{dbl[], dbl[]})  [unwired: 1 in]
      n284 = Add(x=w160, y=w159) -> (x+y=w158:dbl)
      n285 = Add(x=w182, y=w181) -> (x+y=w179:dbl)
      n286 = Divide(x=w158, y=2.0) -> (x/y=w128:dbl)
      "RMS Left" <- w128
      "LeftMovingAvg" <- w128
      n287 = Divide(x=w179, y=2.0) -> (x/y=w129:dbl)
      "RMS Right" <- w129
      "RightMovingAvg" <- w129
      n288 = Build Array(w161, w171) -> (→"2d target":cluster{dbl[], dbl[]}[])
      n289 = Add(x=w128, y=w129) -> (x+y=w177:dbl)
      n290 = Divide(x=w177, y=2.0) -> (x/y=w175:dbl)
      n291 = local write "combined y value"(w175) -> ()
    }
    n292 = local write "Reset Data Acquisition\nAnd UI Updating"("End Program") -> ()
    "Bufffer Index" <- 0.0 ("Bufffer Index")
  }
  "Trial In Progress" <- FALSE ("Trial In Progress")
  "Acquiring Max" <- FALSE ("Acquiring Max")
